vi "SHA256 Hash.vi"(8 "error in":errorcluster, 11 "String":string) -> (0 "error out":errorcluster, 2 "hash":string)   [LabVIEW 2018, in "Password Protection.lvlib"]
uses:
  Password Protection.lvlib
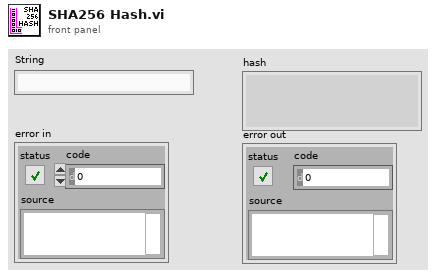
[diagram p1: front panel]
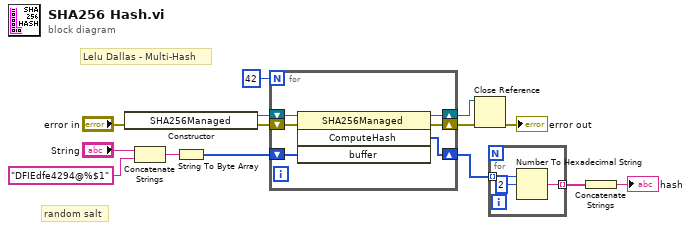
[diagram p0: block diagram]
diagram:
  # "Lelu Dallas - Multi-Hash"
  # "random salt"
  n1 = constructor class="SHA256Managed"(error in="error in") -> (reference out=w14:refnum<k24>, error out=w10:errorcluster)  [unwired: 2 in, 1 out]
  n2 = Concatenate Strings("String", "DFIEdfe4294@%$1" ("string")) -> (w1:string)
  n3 = String To Byte Array(string=w1) -> (unsigned byte array=w13:u8[])
  n4 = for {
    N: 42 -> [_]
    shift-right: [w17] -> w11
    shift-left: w14 -> [w20]
    shift-right: [w15] -> w7
    shift-left: w13 -> [w19]
    shift-right: [w18] -> w12
    shift-left: w10 -> [w16]
    n5 = invoke class="SHA256Managed" method="ComputeHash"(reference=w20, error in=w16, "buffer"=w19) -> (reference out=w17:refnum<k24>, error out=w18:errorcluster, "ComputeHash"=w15:u8[])  [unwired: 1 in, 1 out]
  }
  n6 = Close Reference(reference=w11, error in (no error)=w12) -> (error out=→"error out":errorcluster)
  n7 = for {
    tunnel: w7 -> [w23] mode=indexing
    tunnel: [w22] -> w6 mode=indexing
    n8 = Number To Hexadecimal String(1:i16 2 ("width (-)"), 2:w23) -> (0:w22:string)
  }
  n9 = Concatenate Strings(w6) -> (→"hash":string)
